vi "Eval Polar to Rect Optimal Step.vi"(4 "number of points":u32=10, 5 "radius as function of angle":string, 6 "end":dbl=1.0 format="%.2f", 7 "start":dbl format="%.2f", 8 "epsilon":dbl=0.05 min=1e-18 format="%.2f") -> (0 "error":i32, 1 "ticks":u32, 2 "Y":dbl[](array[numeric]) format="%.2f", 3 "X":dbl[](array[numeric]) format="%.2f")   [LabVIEW 2017, in "NI_Gmath.lvlib"]
doc: "Operates like the Eval Polar to Rect VI but with a significantly higher degree of accuracy."
uses:
  NI_Gmath.lvlib
panel:
  # "Example:\n\n number of points: 100 \n epsilon: 0.05\n start: 0.0\n end: 1.0\n radius as function of angle: t*t+exp(-t)"
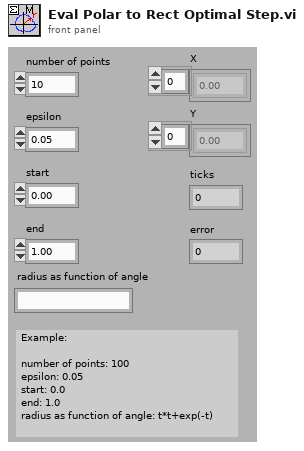
[diagram p1: front panel]
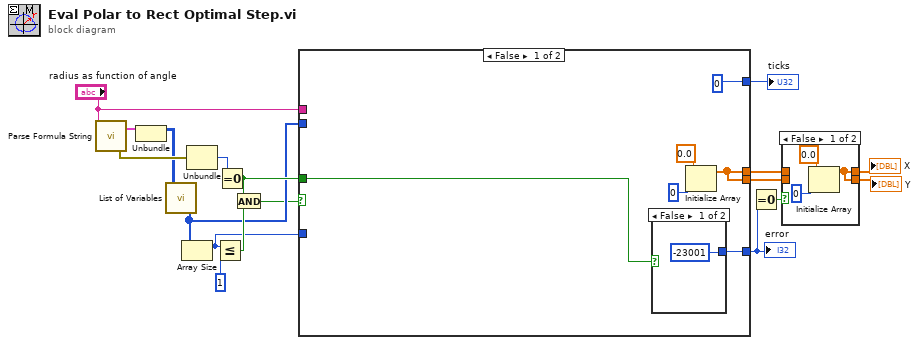
[diagram p0: block diagram]
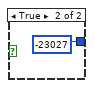
[diagram p3: hidden frame]
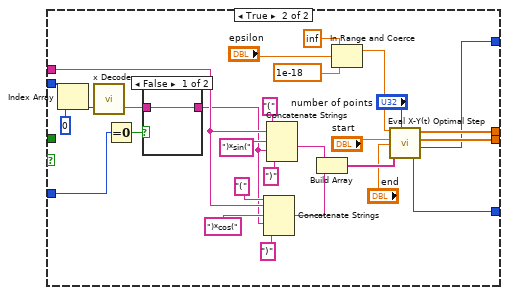
[diagram p4: hidden frame]
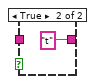
[diagram p5: hidden frame]
diagram:
  n1 = call "Parse Formula String.vi"("formula"="radius as function of angle") -> ("error out"=w16:errorcluster, "Parsed Formula"=w2:cluster{"Table":i32[][], "Y Values":dbl[]})  [unwired: 1 in]
  n2 = Unbundle(w2) -> ("Table"=w1:i32[][])  [unwired: 1 out]
  n3 = call "List of Variables.vi"("Table"=w1) -> ("List of variables"=w12:i32[])
  n4 = Array Size(array=w12) -> (size(s)=w3:i32)
  n5 = Unbundle(w16) -> ("code"=w14:i32)  [unwired: 2 out]
  n6 = Less Or Equal?(x=w3, y=1) -> (x <= y?=w15:bool)
  n7 = Equal To 0?(x=w14) -> (x = 0?=w18:bool)
  n8 = And(x=w18, y=w15) -> (x .and. y?=w11:bool)
  n9 = case shown="False" w11 {
    tunnel: "radius as function of angle" -> [_ w54]
    tunnel: [w20 w49] -> w6
    tunnel: [w20 w48] -> w8
    tunnel: w12 -> [_ w40]
    tunnel: [w23 w38] -> w10
    tunnel: w18 -> [w24 _]
    tunnel: [u32 0 w37] -> w4
    tunnel: w3 -> [_ w34]
    frame False {
      n10 = case shown="False" w24 {
        tunnel: [-23001 -23027] -> w23
        frame False {
        }
        frame True {
        }
      }
      n11 = Initialize Array(0.0, 0) -> (w20:dbl[])
    }
    frame True {
      n12 = Index Array(array=w40, index=0) -> (element=w39:i32)
      n13 = call "x Decode.vi"("number"=w39) -> ("x string"=w32:string)  [unwired: 1 in, 1 out]
      n14 = Equal To 0?(x=w34) -> (x = 0?=w33:bool)
      n15 = case shown="False" w33 {
        tunnel: w32 -> [w55 _]
        tunnel: [w55 "t"] -> w31
        frame False {
        }
        frame True {
        }
      }
      n16 = Concatenate Strings("(", w54, ")*cos(", w31, ")") -> (w47:string)
      n17 = Concatenate Strings("(", w54, ")*sin(", w31, ")") -> (w46:string)
      n18 = Build Array(w46, w47) -> (w53:string[])
      n19 = In Range and Coerce(upper limit=inf, x="epsilon", lower limit=1e-18) -> (coerced(x)=w30:dbl)  [unwired: 1 out]
      n20 = call "Eval X-Y(t) Optimal Step.vi"("number of points"="number of points", "Formulas"=w53, "end"="end", "start"="start", "epsilon"=w30) -> ("error"=w38:i32, "ticks"=w37:u32, "Y"=w49:dbl[], "X"=w48:dbl[])
    }
  }
  "error" <- w10
  "ticks" <- w4
  n21 = Equal To 0?(x=w10) -> (x = 0?=w9:bool)
  n22 = case shown="False" w9 {
    tunnel: w8 -> [_ w61]
    tunnel: [w57 w61] -> w7
    tunnel: w6 -> [_ w60]
    tunnel: [w57 w60] -> w5
    frame False {
      n23 = Initialize Array(0.0, 0) -> (w57:dbl[])
    }
    frame True {
    }
  }
  "X" <- w7
  "Y" <- w5
